vi "BFS Find Neighbors.vi"(1 "Coordinate (0, 0)":T1, 2 "Visited":bool[][](array[boolean]), 3 "Data":bool[][](array[boolean])) -> (0 "Connected Neighbors":T1[](array[typedef]))   [LabVIEW 2018, in "Video Cam Processor.lvclass"]
uses:
  Video Cam Processor.lvclass
  Private/Hull Point STYP.ctl
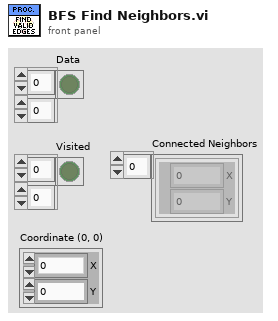
[diagram p1: front panel]
types:
  T1 = typedef "Video Cam Processor.lvclass/Hull Point STYP.ctl" = cluster{"X":i32, "Y":i32}
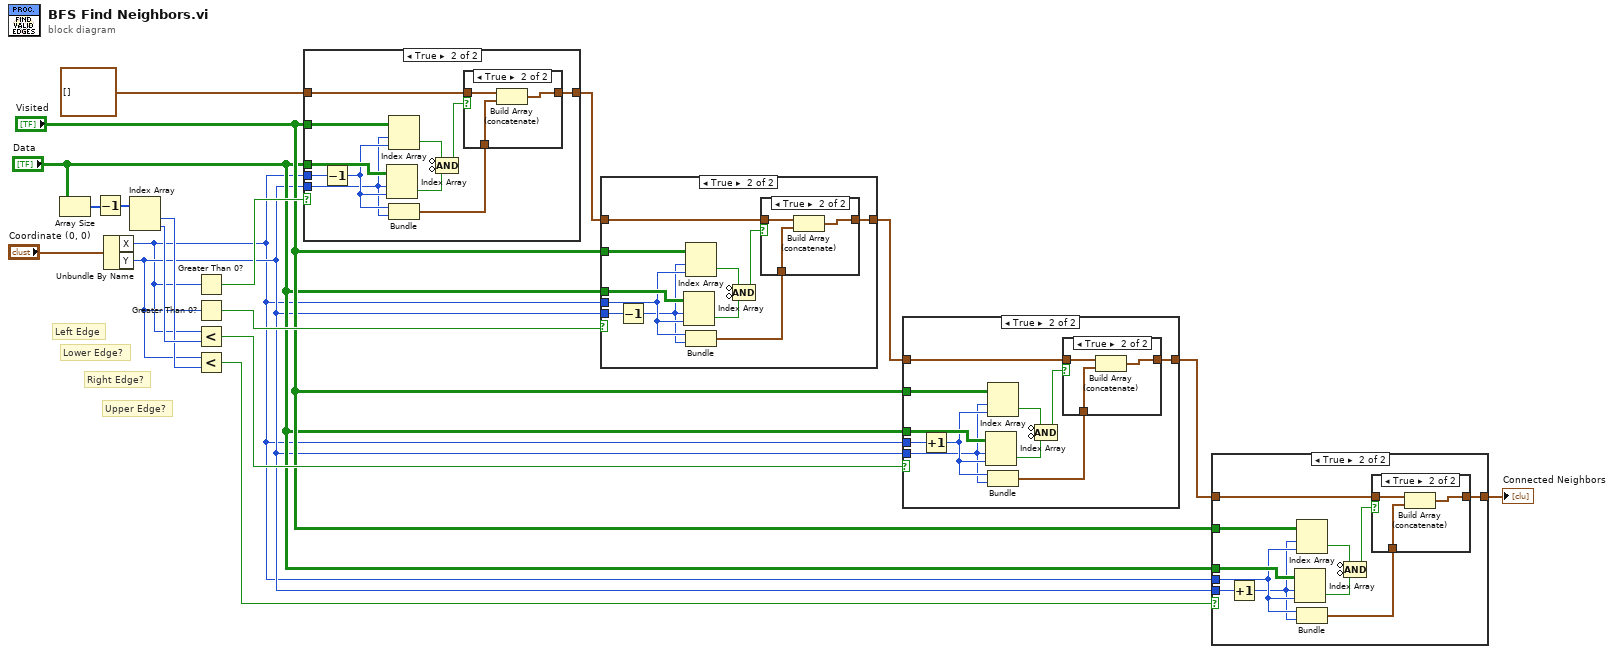
[diagram p0: block diagram]
diagram:
  # "Left Edge"
  # "Right Edge?"
  # "Upper Edge?"
  # "Lower Edge?"
  n1 = Array Size(array="Data") -> (size(s)=w16:i32[])
  n2 = Decrement(x=w16) -> (x-1=w17:i32[])
  n3 = Unbundle By Name("Coordinate (0, 0)") -> ("X"=w1:i32, "Y"=w4:i32)
  n4 = Index Array(array=w17) -> (element #1=w14:i32, element #2=w15:i32)  [unwired: 2 in]
  n5 = Greater Than 0?(x=w1) -> (x > 0?=w13:bool)
  n6 = Greater Than 0?(x=w4) -> (x > 0?=w10:bool)
  n7 = Less?(x=w1, y=w15) -> (x < y?=w8:bool)
  n8 = Less?(x=w4, y=w14) -> (x < y?=w3:bool)
  n9 = case shown="True" w13 {
    tunnel: "Visited" -> [_ w28]
    tunnel: "Data" -> [_ w30]
    tunnel: w1 -> [_ w29]
    tunnel: w4 -> [_ w22]
    tunnel: T1[] [] ("Connected Neighbors") -> [w19 w24]
    tunnel: [w19 w20] -> w11
    frame False {
    }
    frame True {
      n10 = Decrement(x=w29) -> (x-1=w23:i32)
      n11 = Index Array(array=w30, index (row)=w22, index (col)=w23) -> (element=w26:bool)
      n12 = Index Array(array=w28, index (row)=w22, index (col)=w23) -> (element=w27:bool)
      n13 = Bundle(w23, "Y"=w22) -> (w21:cluster{i32, "Y":i32})  [unwired: 1 in]
      n14 = Compound Arithmetic op=AND(invert w27, invert w26) -> (w25:bool)
      n15 = case shown="True" w25 {
        tunnel: w24 -> [w31 w34]
        tunnel: w21 -> [_ w33]
        tunnel: [w31 w32] -> w20
        frame False {
        }
        frame True {
          n16 = Build Array (concatenate)(w34, w33) -> (w32:T1[])
        }
      }
    }
  }
  n17 = case shown="True" w10 {
    tunnel: "Visited" -> [_ w45]
    tunnel: "Data" -> [_ w46]
    tunnel: w1 -> [_ w37]
    tunnel: w4 -> [_ w40]
    tunnel: w11 -> [w35 w41]
    tunnel: [w35 w38] -> w9
    frame False {
    }
    frame True {
      n18 = Decrement(x=w40) -> (x-1=w36:i32)
      n19 = Index Array(array=w46, index (row)=w36, index (col)=w37) -> (element=w43:bool)
      n20 = Index Array(array=w45, index (row)=w36, index (col)=w37) -> (element=w44:bool)
      n21 = Bundle("X"=w37, w36) -> (w39:cluster{"X":i32, i32})  [unwired: 1 in]
      n22 = Compound Arithmetic op=AND(invert w44, invert w43) -> (w42:bool)
      n23 = case shown="True" w42 {
        tunnel: w41 -> [w47 w50]
        tunnel: w39 -> [_ w49]
        tunnel: [w47 w48] -> w38
        frame False {
        }
        frame True {
          n24 = Build Array (concatenate)(w50, w49) -> (w48:T1[])
        }
      }
    }
  }
  n25 = case shown="True" w8 {
    tunnel: "Visited" -> [_ w60]
    tunnel: "Data" -> [_ w62]
    tunnel: w1 -> [_ w61]
    tunnel: w4 -> [_ w54]
    tunnel: w9 -> [w51 w56]
    tunnel: [w51 w52] -> w7
    frame False {
    }
    frame True {
      n26 = Increment(x=w61) -> (x+1=w55:i32)
      n27 = Index Array(array=w62, index (row)=w54, index (col)=w55) -> (element=w58:bool)
      n28 = Index Array(array=w60, index (row)=w54, index (col)=w55) -> (element=w59:bool)
      n29 = Bundle(w55, "Y"=w54) -> (w53:cluster{i32, "Y":i32})  [unwired: 1 in]
      n30 = Compound Arithmetic op=AND(invert w59, invert w58) -> (w57:bool)
      n31 = case shown="True" w57 {
        tunnel: w56 -> [w63 w66]
        tunnel: w53 -> [_ w65]
        tunnel: [w63 w64] -> w52
        frame False {
        }
        frame True {
          n32 = Build Array (concatenate)(w66, w65) -> (w64:T1[])
        }
      }
    }
  }
  n33 = case shown="True" w3 {
    tunnel: "Visited" -> [_ w77]
    tunnel: "Data" -> [_ w78]
    tunnel: w1 -> [_ w69]
    tunnel: w4 -> [_ w72]
    tunnel: w7 -> [w67 w73]
    tunnel: [w67 w70] -> w2
    frame False {
    }
    frame True {
      n34 = Increment(x=w72) -> (x+1=w68:i32)
      n35 = Index Array(array=w78, index (row)=w68, index (col)=w69) -> (element=w75:bool)
      n36 = Index Array(array=w77, index (row)=w68, index (col)=w69) -> (element=w76:bool)
      n37 = Bundle("X"=w69, w68) -> (w71:cluster{"X":i32, i32})  [unwired: 1 in]
      n38 = Compound Arithmetic op=AND(invert w76, invert w75) -> (w74:bool)
      n39 = case shown="True" w74 {
        tunnel: w73 -> [w79 w82]
        tunnel: w71 -> [_ w81]
        tunnel: [w79 w80] -> w70
        frame False {
        }
        frame True {
          n40 = Build Array (concatenate)(w82, w81) -> (w80:T1[])
        }
      }
    }
  }
  "Connected Neighbors" <- w2
